vi "Compile Channel Group Refs.vi"(8 "error in":errorcluster, 11 "Channel Groups in":T3(array[cluster]) {"Channel Data References" format="%.0x"}) -> (0 "error out":errorcluster, 3 "CompiledChannelGroupings":T1)   [LabVIEW 2026, in "SystemMonitor Deployment Hooks.lvlib"]
uses:
  SystemMonitor Deployment Hooks.lvlib
  Shared/GroupedChannelRefs.ctl
  Types/Channel Mode.ctl
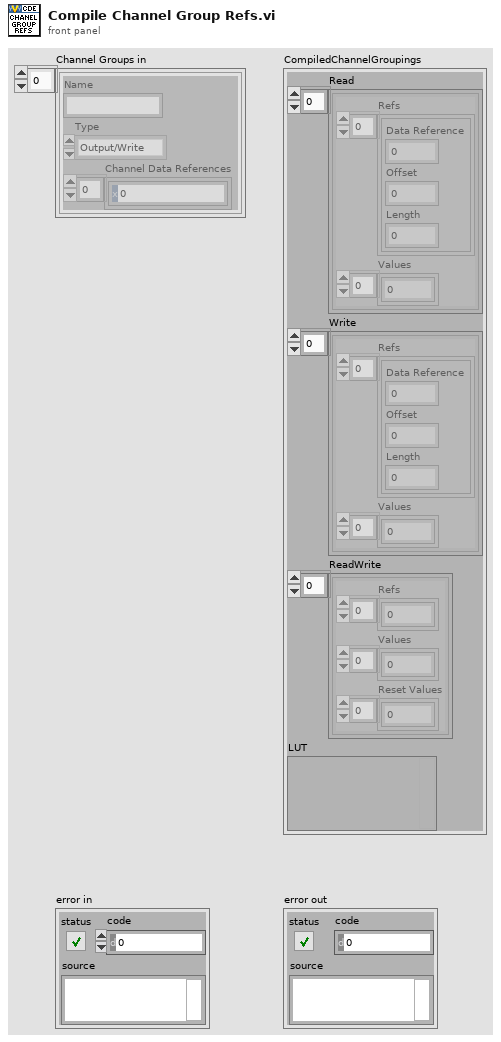
[diagram p1: front panel]
types:
  T1 = typedef "GroupedChannelRefs.ctl" = cluster{"Read":cluster{"Refs":cluster{"Data Reference":i32, "Offset":u64, "Length":u64}[], "Values":dbl[]}[], "Write":cluster{"Refs":cluster{"Data Reference":i32, "Offset":u64, "Length":u64}[], "Values":dbl[]}[], "ReadWrite":cluster{"Refs":i32[], "Values":dbl[], "Reset Values":dbl[]}[], "LUT":variant}
  T2 = typedef "SystemMonitor Deployment Hooks.lvlib/Channel Mode.ctl" = enum16{"Output/Write", "Input/Read", "Input/ReadWrite"}
  T3 = cluster{"Name":string, "Type":T2, "Channel Data References":i32[]}[]
  T4 = cluster{"Refs":cluster{"Data Reference":i32, "Offset":u64, "Length":u64}[], "Values":dbl[]}[]
  T5 = cluster{"Refs":i32[], "Values":dbl[], "Reset Values":dbl[]}[]
  T6 = cluster{"Refs":cluster{"Data Reference":i32, "Offset":u64, "Length":u64}[], "Values":dbl[]}
  T7 = cluster{"Refs":i32[], "Values":dbl[], "Reset Values":dbl[]}
  T8 = cluster{"Data Reference":i32, "Offset":u64, "Length":u64}[]
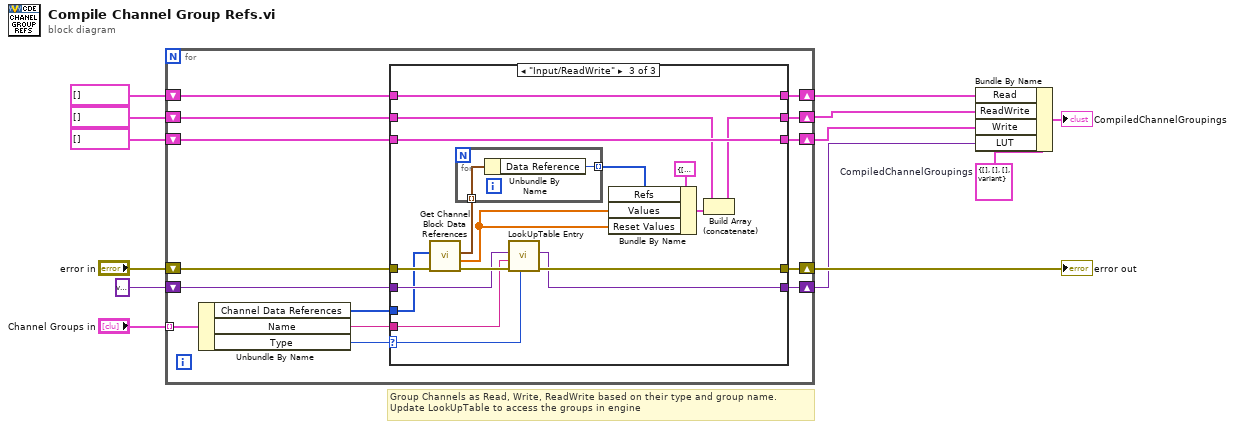
[diagram p0: block diagram]
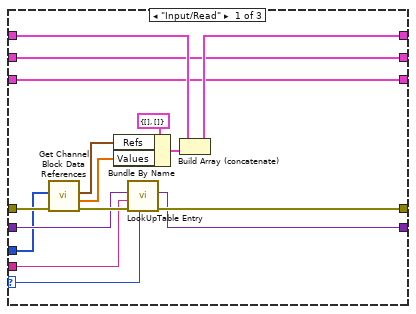
[diagram p2: hidden frame]
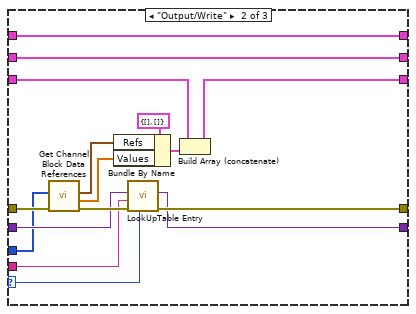
[diagram p3: hidden frame]
diagram:
  w10 = T1 {"Read"=[], "Write"=[], "ReadWrite"=[], "LUT"=variant}  # CompiledChannelGroupings
  # "Group Channels as Read, Write, ReadWrite based on their type and group name. \nUpdate LookUpTable to access the groups in engine"
  n1 = for {
    tunnel: "Channel Groups in" -> [w25] mode=indexing
    shift-right: [w26] -> w12
    shift-left: "error in" -> [w27]
    shift-right: [w22] -> w2
    shift-left: variant ("LUT") -> [w23]
    shift-right: [w21] -> w4
    shift-left: T4 [] -> [w16]
    shift-right: [w18] -> w3
    shift-left: T5 [] -> [w17]
    shift-right: [w15] -> w5
    shift-left: T4 [] -> [w14]
    n2 = Unbundle By Name(w25) -> ("Channel Data References"=w24:i32[], "Name"=w20:string, "Type"=w19:T2)
    n3 = case shown="\"Input/ReadWrite\"" w19 {
      selector: w19 -> [w39 w55 w73]
      tunnel: w27 -> [w42 w58 w75]
      tunnel: [w43 w59 w76] -> w26
      tunnel: w24 -> [w28 w47 w68]
      tunnel: w23 -> [w32 w51 w70]
      tunnel: [w31 w50 w69] -> w22
      tunnel: [w36 w46 w67] -> w21
      tunnel: w20 -> [w33 w52 w71]
      tunnel: [w35 w53 w65] -> w18
      tunnel: w17 -> [w35 w53 w64]
      tunnel: w16 -> [w38 w46 w67]
      tunnel: [w34 w45 w66] -> w15
      tunnel: w14 -> [w34 w44 w66]
      frame "Input/Read" {
        n4 = call "Get Channel Block Data References.vi"("error in"=w42, "Channel Data Refs"=w28) -> ("error out"=w41:errorcluster, "Values Array"=w29:dbl[], "Block Data Refs"=w30:T8)  [unwired: 7 in]
        n5 = Bundle By Name(cluster=T6 {"Refs"=[], "Values"=[]}, "Refs"=w30, "Values"=w29) -> (w37:T6)
        n6 = call "LookUpTable Entry.vi"("Type"=w39, "error in"=w41, "Name"=w33, "LUT"=w32) -> ("error out"=w43:errorcluster, "LUT"=w31:variant)  [unwired: 6 in]
        n7 = Build Array (concatenate)(w38, w37) -> (w36:T4)
      }
      frame "Output/Write" {
        n8 = call "Get Channel Block Data References.vi"("error in"=w58, "Channel Data Refs"=w47) -> ("error out"=w57:errorcluster, "Values Array"=w48:dbl[], "Block Data Refs"=w49:T8)  [unwired: 7 in]
        n9 = Bundle By Name(cluster=T6 {"Refs"=[], "Values"=[]}, "Refs"=w49, "Values"=w48) -> (w54:T6)
        n10 = call "LookUpTable Entry.vi"("Type"=w55, "error in"=w57, "Name"=w52, "LUT"=w51) -> ("error out"=w59:errorcluster, "LUT"=w50:variant)  [unwired: 6 in]
        n11 = Build Array (concatenate)(w44, w54) -> (w45:T4)
      }
      frame "Input/ReadWrite" {
        n12 = call "Get Channel Block Data References.vi"("error in"=w75, "Channel Data Refs"=w68) -> ("error out"=w74:errorcluster, "Values Array"=w62:dbl[], "Block Data Refs"=w61:T8)  [unwired: 7 in]
        n13 = for {
          tunnel: w61 -> [w78] mode=indexing
          tunnel: [w77] -> w60 mode=indexing
          n14 = Unbundle By Name(w78) -> ("Data Reference"=w77:i32)
        }
        n15 = call "LookUpTable Entry.vi"("Type"=w73, "error in"=w74, "Name"=w71, "LUT"=w70) -> ("error out"=w76:errorcluster, "LUT"=w69:variant)  [unwired: 6 in]
        n16 = Bundle By Name(cluster=T7 {"Refs"=[], "Values"=[], "Reset Values"=[]}, "Refs"=w60, "Values"=w62, "Reset Values"=w62) -> (w72:T7)
        n17 = Build Array (concatenate)(w64, w72) -> (w65:T5)
      }
    }
  }
  "error out" <- w12
  n18 = Bundle By Name(cluster=w10, "Read"=w4, "ReadWrite"=w3, "Write"=w5, "LUT"=w2) -> (→"CompiledChannelGroupings":T1)
